vi "Copy.vi"(0 "Case Structure in":refnum<class "Case Structure.lvclass">, 1 "Linked List Ref":refnum<data-value>, 2 "New Parent ID":string, 5 "Test ID":string, 7 "Insertion Index":i32=-1, 9 "Move?":bool, 11 "error in (no error)":errorcluster, 12 "New ID":string, 13 "Data IDs":variant) -> (3 "Linked List Ref out":refnum<data-value>, 6 "Linked List ID out":string, 14 "Data IDs out":variant, 15 "error out":errorcluster)   [LabVIEW 2017, in "Test Executive.lvlib" / "Case Structure.lvclass"]
uses:
  <vilib>/gpm_packages/@cs/test-executive/Source/Test Executive/Case Structure/Case Structure.lvclass
  <vilib>/gpm_packages/@cs/linked-list/Source/Linked List/ILinkedList/ILinked List.lvclass
  <vilib>/gpm_packages/@cs/test-executive/Source/Test Executive/Executioner/Executioner.lvclass
  170d0bf8-3ce4-4b61-beee-8de6a9555dcd.vi
  8c6f9ea9-cb7b-4d30-8c6c-37deb1dc3811.vi
  32fd4f95-6d36-497c-8072-1c0c73e647a5.vi
  b738481c-fbd3-4aec-95cc-cf1e4be5b944.vi
  d1639552-7065-4fb1-b1e9-68cb85843caa.vi
  6d937740-c15e-44ca-94b0-4320c414bdba.vi
  439bdb0e-a58c-4a1e-b65e-cefac105e484.vi
  28a4d2c3-02d8-45de-ad56-a7f6d6817309.vi
  <vilib>/gpm_packages/@cs/linked-list/Source/Linked List/Linked List Ref/Linked List Ref.lvclass
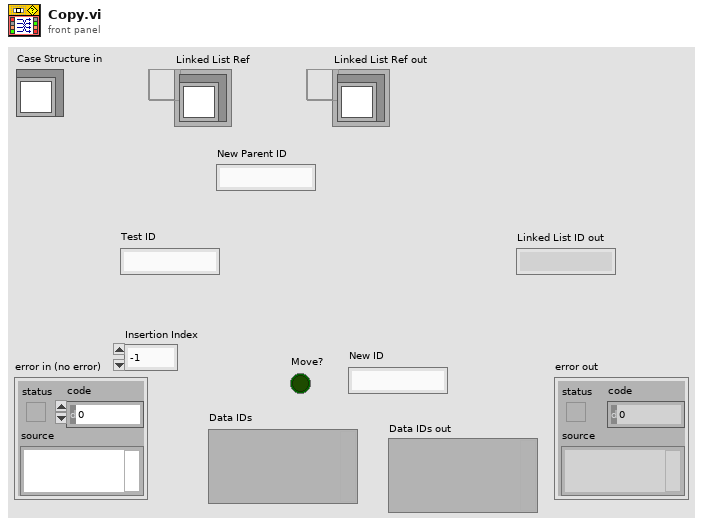
[diagram p1: front panel]
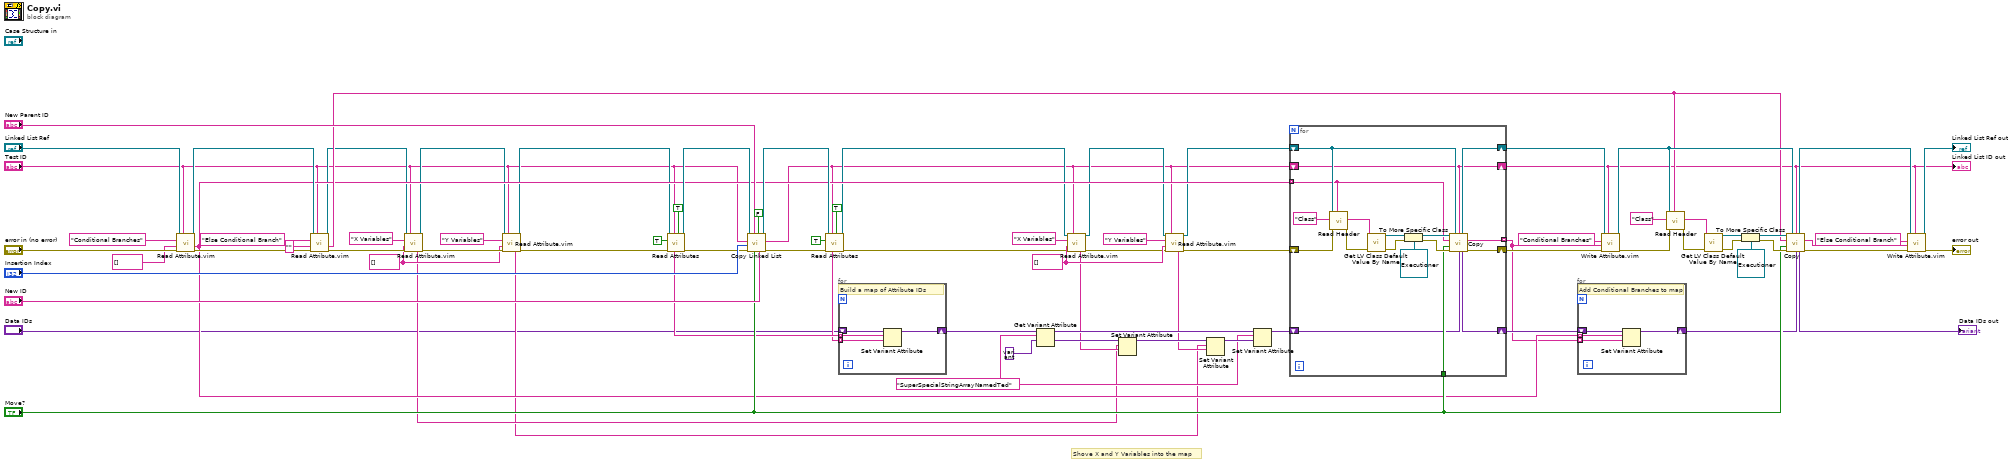
[diagram p0: block diagram]
diagram:
  w22 = "SuperSpecialStringArrayNamedTed" ("name")
  w17 = string[] []
  w26 = string[] []
  # "Shove X and Y Variables into the map"
  n1 = call "Read Attribute.vim"("Linked List Ref"="Linked List Ref", "Linked List ID"="Test ID", "Attribute Name"="Conditional Branches", "Type"=string[] [], "error in (no error)"="error in (no error)") -> ("Linked List Ref out"=w72:refnum<data-value>, "Attribute"=w38:string[], "error out"=w73:errorcluster)  [unwired: 5 in, 3 out]
  n2 = call "Read Attribute.vim"("Linked List Ref"=w72, "Linked List ID"="Test ID", "Attribute Name"="Else Conditional Branch", "Type"="", "error in (no error)"=w73) -> ("Linked List Ref out"=w32:refnum<data-value>, "Attribute"=w51:string, "error out"=w34:errorcluster)  [unwired: 5 in, 3 out]
  n3 = call "Read Attribute.vim"("Linked List Ref"=w32, "Linked List ID"="Test ID", "Attribute Name"="X Variables", "Type"=w26, "error in (no error)"=w34) -> ("Linked List Ref out"=w31:refnum<data-value>, "Data ID"=w5:string, "error out"=w35:errorcluster)  [unwired: 5 in, 3 out]
  n4 = call "Read Attribute.vim"("Linked List Ref"=w31, "Linked List ID"="Test ID", "Attribute Name"="Y Variables", "Type"=w26, "error in (no error)"=w35) -> ("Linked List Ref out"=w30:refnum<data-value>, "Data ID"=w4:string, "error out"=w33:errorcluster)  [unwired: 5 in, 3 out]
  n5 = call <vilib>:"Read Attributes.vi"("Flatten Pointer?"=TRUE, "Linked List ID"="Test ID", "error in (no error)"=w33, "Include Private?"=TRUE, "Linked List Ref"=w30) -> ("error out"=w42:errorcluster, "Linked List Ref out"=w41:refnum<data-value>, "Data IDs"=w25:string[])  [unwired: 1 in, 3 out]
  n6 = call <vilib>:"Copy Linked List.vi"("New Linked List ID"="New ID", "Recursive? (T)"=FALSE, "Move?"="Move?", "New Parent Linked List ID"="New Parent ID", "error in (no error)"=w42, "Insertion Index"="Insertion Index", "Linked List ID"="Test ID", "Linked List Ref"=w41) -> ("error out"=w46:errorcluster, "Linked List ID out"=w6:string, "Linked List Ref out"=w45:refnum<data-value>)  [unwired: 1 out]
  n7 = call <vilib>:"Read Attributes.vi"("Flatten Pointer?"=TRUE, "Linked List ID"=w6, "error in (no error)"=w46, "Include Private?"=TRUE, "Linked List Ref"=w45) -> ("error out"=w13:errorcluster, "Linked List Ref out"=w9:refnum<data-value>, "Data IDs"=w24:string[])  [unwired: 1 in, 3 out]
  n8 = for {
    tunnel: w25 -> [w85] mode=indexing
    tunnel: w24 -> [w84] mode=indexing
    shift-right: [w83] -> w2
    shift-left: "Data IDs" -> [w86]
    # "Build a map of Attribute IDs"
    n9 = Set Variant Attribute(Variant=w86, name=w85, value=w84) -> (Variant out=w83:variant)  [unwired: 1 in, 2 out]
  }
  n10 = Get Variant Attribute(Variant=w2, name=w22, default value (empty Variant)=variant ("default value (empty variant)")) -> (duplicate Variant=w21:variant, value=w19:variant)  [unwired: 1 in, 2 out]
  n11 = call "Read Attribute.vim"("Linked List Ref"=w9, "Linked List ID"=w6, "Attribute Name"="X Variables", "Type"=w17, "error in (no error)"=w13) -> ("Linked List Ref out"=w8:refnum<data-value>, "Data ID"=w11:string, "error out"=w14:errorcluster)  [unwired: 5 in, 3 out]
  n12 = Set Variant Attribute(Variant=w19, name=w5, value=w11) -> (Variant out=w20:variant)  [unwired: 1 in, 2 out]
  n13 = call "Read Attribute.vim"("Linked List Ref"=w8, "Linked List ID"=w6, "Attribute Name"="Y Variables", "Type"=w17, "error in (no error)"=w14) -> ("Linked List Ref out"=w7:refnum<data-value>, "Data ID"=w10:string, "error out"=w12:errorcluster)  [unwired: 5 in, 3 out]
  n14 = Set Variant Attribute(Variant=w20, name=w4, value=w10) -> (Variant out=w23:variant)  [unwired: 1 in, 2 out]
  n15 = Set Variant Attribute(Variant=w21, name=w22, value=w23) -> (Variant out=w1:variant)  [unwired: 1 in, 2 out]
  n16 = for {
    tunnel: "Move?" -> [w92]
    tunnel: w38 -> [w91] mode=indexing
    shift-right: [w94] -> w71
    shift-left: w12 -> [w96]
    shift-right: [w93] -> w69
    shift-left: w7 -> [w95]
    shift-right: [w90] -> w49
    shift-left: w6 -> [w90]
    tunnel: [w89] -> w37 mode=indexing
    shift-right: [w87] -> w40
    shift-left: w1 -> [w88]
    n17 = call <vilib>:"Read Header.vi"("Linked List ID"=w91, "error in (no error)"=w96, "Header Name"="Class", "Linked List Ref"=w95) -> ("error out"=w101:errorcluster, "Header Value"=w103:string)  [unwired: 4 in, 2 out]
    n18 = call <vilib>:"Get LV Class Default Value By Name.vi"("error in (no error)"=w101, "class name"=w103) -> ("error out"=w100:errorcluster, "object"=w102:refnum<class>)  [unwired: 8 in]
    n19 = To More Specific Class(target class=refnum<class "Executioner.lvclass"> refnum ("Test Executive.lvlib:Executioner.lvclass"), reference=w102, error in=w100) -> (specific class reference=w97:refnum<class "Executioner.lvclass">, error out=w98:errorcluster)
    n20 = call-dynamic "Copy.vi"("Executioner in"=w97, "Linked List Ref"=w95, "New Parent ID"=w90, "Test ID"=w91, "Move?"=w92, "error in (no error)"=w98, "Data IDs"=w88) -> ("Linked List Ref out"=w93:refnum<data-value>, "Linked List ID out"=w89:string, "Data IDs out"=w87:variant, "error out"=w94:errorcluster)  [unwired: 5 in]
  }
  "Linked List ID out" <- w49
  n21 = for {
    tunnel: w38 -> [w107] mode=indexing
    tunnel: w37 -> [w106] mode=indexing
    shift-right: [w105] -> w39
    shift-left: w40 -> [w108]
    # "Add Conditional Branches to map"
    n22 = Set Variant Attribute(Variant=w108, name=w107, value=w106) -> (Variant out=w105:variant)  [unwired: 1 in, 2 out]
  }
  n23 = call "Write Attribute.vim"("Linked List ID"=w49, "error in (no error)"=w71, "Attribute"=w37, "Attribute Name"="Conditional Branches", "Linked List Ref"=w69) -> ("error out"=w55:errorcluster, "Linked List Ref out"=w56:refnum<data-value>)  [unwired: 3 in, 2 out]
  n24 = call <vilib>:"Read Header.vi"("Linked List ID"=w51, "error in (no error)"=w55, "Header Name"="Class", "Linked List Ref"=w56) -> ("error out"=w60:errorcluster, "Header Value"=w58:string)  [unwired: 4 in, 2 out]
  n25 = call <vilib>:"Get LV Class Default Value By Name.vi"("error in (no error)"=w60, "class name"=w58) -> ("error out"=w61:errorcluster, "object"=w59:refnum<class>)  [unwired: 8 in]
  n26 = To More Specific Class(target class=refnum<class "Executioner.lvclass"> refnum ("Test Executive.lvlib:Executioner.lvclass"), reference=w59, error in=w61) -> (specific class reference=w64:refnum<class "Executioner.lvclass">, error out=w63:errorcluster)
  n27 = call-dynamic "Copy.vi"("Executioner in"=w64, "Linked List Ref"=w56, "New Parent ID"=w49, "Test ID"=w51, "Move?"="Move?", "error in (no error)"=w63, "Data IDs"=w39) -> ("Linked List Ref out"=w68:refnum<data-value>, "Linked List ID out"=w67:string, "Data IDs out"=→"Data IDs out":variant, "error out"=w65:errorcluster)  [unwired: 5 in]
  n28 = call "Write Attribute.vim"("Linked List ID"=w49, "error in (no error)"=w65, "Attribute"=w67, "Attribute Name"="Else Conditional Branch", "Linked List Ref"=w68) -> ("error out"=→"error out":errorcluster, "Linked List Ref out"=→"Linked List Ref out":refnum<data-value>)  [unwired: 3 in, 2 out]
